vi "Write log file.vi"(8 "error in":errorcluster, 10 "UDcluster Array in":T1[](array[typedef]), 11 "file path (use dialog)":path) -> (0 "error out":errorcluster, 3 "path":path)   [LabVIEW 2012]
uses:
  typedef/Log_User_Data.ctl
  typedef/User Accounts.ctl
panel:
  out "Array 3":string[](array[string])
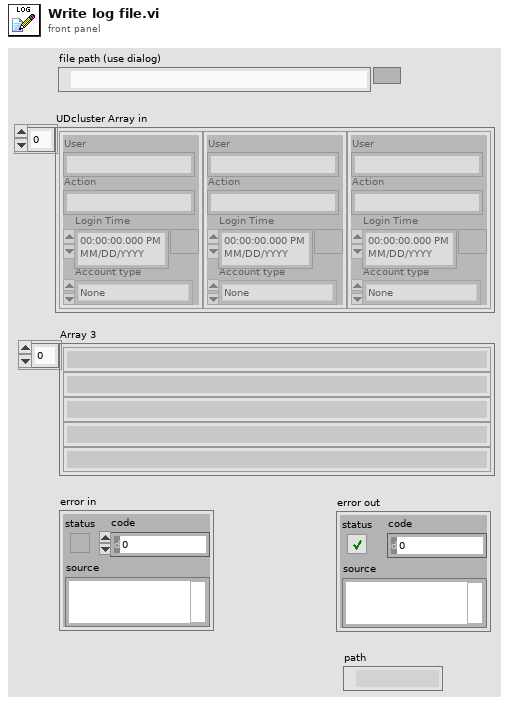
[diagram p1: front panel]
types:
  T1 = typedef "Log_User_Data.ctl" = cluster{"User":string, "Action":string, "Account type":T2, "Login Time ":timestamp}
  T2 = typedef "User Accounts.ctl" = enum16{"None", "User", "Admin"}
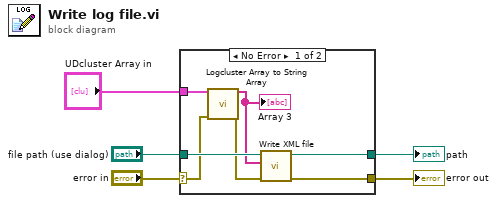
[diagram p0: block diagram]
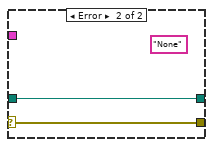
[diagram p2: hidden frame]
diagram:
  n1 = case shown="No Error" "error in" {
    selector: "error in" -> [w7 w14]
    tunnel: "file path (use dialog)" -> [w12 w13]
    tunnel: [w11 w14] -> w4
    tunnel: [w10 w13] -> w3
    tunnel: "UDcluster Array in" -> [w6 _]
    frame No Error {
      n2 = call "Logcluster Array to String Array.vi"("UDcluster Array in"=w6, "error in (no error)"=w7) -> ("UDarray out"=w9:string[], "error out"=w8:errorcluster)  [unwired: 12 in]
      "Array 3" <- w9
      n3 = call "Write XML file.vi"("error in (no error)"=w8, "Array in"=w9, "file path (use dialog)"=w12) -> ("error out"=w11:errorcluster, "path"=w10:path)  [unwired: 6 in, 1 out]
    }
    frame Error {
      (unwired) "None" ("xml string")
    }
  }
  "error out" <- w4
  "path" <- w3
